vi "THD_MSA.vi"() -> ()   [LabVIEW 2012]
panel:
  out "Meas_Error":bool=TRUE
  in  "timeout(s)":dbl=10.0
  out "index":i32=48
  out "mean(THD)":dbl=0.5
  out "Sensitivity(mVeff/Pa)":dbl=336.0
  in  "Std_Deviation_Thresold":dbl=0.04
  in  "Excitation_amplitude(Vpeak)":dbl=0.35 min=0.0 format="%.3f"
  in  "Sound_Pressure(dB SPL)":dbl=94.0502
  in  "stop":bool=TRUE
  in  "Anzahl der Messungen":i32=200
  out "XY Graph":cluster{dbl[], dbl[]}[](graph)=[{[0.84, 0.944, 1.048, 1.1540000000000001, 1.2590000000000001, 1.3650000000000002, 1.4670000000000003, 1.5720000000000003, 1.6750000000000003, 1.7800000000000002, 1.8880000000000003, 1.9940000000000004, 2.0990000000000006, 2.206000000000001, 2.3080000000000007, 2.412000000000001, 2.520000000000001, 2.626000000000001, 2.733000000000001, 2.836000000000001, 2.942000000000001, 3.048000000000001, 3.154000000000001, 3.2600000000000007, 3.3640000000000008, 3.467000000000001, 3.573000000000001, 3.677000000000001, 3.783000000000001, 3.888000000000001, 3.9930000000000008, 4.099000000000001, 4.201000000000001, 4.307000000000001, 4.412000000000002, 4.517000000000002, 4.6220000000000026, 4.721000000000003, 4.827000000000003, 4.9330000000000025, 5.039000000000002, 5.1430000000000025, 5.248000000000003, 5.354000000000003, 5.461000000000003, 5.568000000000003, 5.674000000000003, 5.780000000000003, 5.885000000000003], [0.5, 0.5, 0.5, 0.5, 0.5, 0.5, 0.5, 0.5, 0.5, 0.5, 0.5, 0.5, 0.5, 0.5, 0.5, 0.5, 0.5, 0.5, 0.5, 0.5, 0.5, 0.5, 0.5, 0.5, 0.5, 0.5, 0.5, 0.5, 0.5, 0.5, 0.5, 0.5, 0.5, 0.5, 0.5, 0.5, 0.5, 0.5, 0.5, 0.5, 0.5, 0.5, 0.5, 0.5, 0.5, 0.5, 0.5, 0.5, 0.5]}, {[0.84, 0.944, 1.048, 1.1540000000000001, 1.2590000000000001, 1.3650000000000002, 1.4670000000000003, 1.5720000000000003, 1.6750000000000003, 1.7800000000000002, 1.8880000000000003, 1.9940000000000004, 2.0990000000000006, 2.206000000000001, 2.3080000000000007, 2.412000000000001, 2.520000000000001, 2.626000000000001, 2.733000000000001, 2.836000000000001, 2.942000000000001, 3.048000000000001, 3.154000000000001, 3.2600000000000007, 3.3640000000000008, 3.467000000000001, 3.573000000000001, 3.677000000000001, 3.783000000000001, 3.888000000000001, 3.9930000000000008, 4.099000000000001, 4.201000000000001, 4.307000000000001, 4.412000000000002, 4.517000000000002, 4.6220000000000026, 4.721000000000003, 4.827000000000003, 4.9330000000000025, 5.039000000000002, 5.1430000000000025, 5.248000000000003, 5.354000000000003, 5.461000000000003, 5.568000000000003, 5.674000000000003, 5.780000000000003, 5.885000000000003], [336.0, 336.0, 336.0, 336.0, 336.0, 336.0, 336.0, 336.0, 336.0, 336.0, 336.0, 336.0, 336.0, 336.0, 336.0, 336.0, 336.0, 336.0, 336.0, 336.0, 336.0, 336.0, 336.0, 336.0, 336.0, 336.0, 336.0, 336.0, 336.0, 336.0, 336.0, 336.0, 336.0, 336.0, 336.0, 336.0, 336.0, 336.0, 336.0, 336.0, 336.0, 336.0, 336.0, 336.0, 336.0, 336.0, 336.0, 336.0, 336.0]}, {[0.84, 0.944, 1.048, 1.1540000000000001, 1.2590000000000001, 1.3650000000000002, 1.4670000000000003, 1.5720000000000003, 1.6750000000000003, 1.7800000000000002, 1.8880000000000003, 1.9940000000000004, 2.0990000000000006, 2.206000000000001, 2.3080000000000007, 2.412000000000001, 2.520000000000001, 2.626000000000001, 2.733000000000001, 2.836000000000001, 2.942000000000001, 3.048000000000001, 3.154000000000001, 3.2600000000000007, 3.3640000000000008, 3.467000000000001, 3.573000000000001, 3.677000000000001, 3.783000000000001, 3.888000000000001, 3.9930000000000008, 4.099000000000001, 4.201000000000001, 4.307000000000001, 4.412000000000002, 4.517000000000002, 4.6220000000000026, 4.721000000000003, 4.827000000000003, 4.9330000000000025, 5.039000000000002, 5.1430000000000025, 5.248000000000003, 5.354000000000003, 5.461000000000003, 5.568000000000003, 5.674000000000003, 5.780000000000003, 5.885000000000003], [0.84, 0.104, 0.104, 0.106, 0.105, 0.106, 0.102, 0.105, 0.103, 0.105, 0.108, 0.106, 0.105, 0.107, 0.102, 0.104, 0.108, 0.106, 0.107, 0.103, 0.106, 0.106, 0.106, 0.106, 0.104, 0.103, 0.106, 0.104, 0.106, 0.105, 0.105, 0.106, 0.102, 0.106, 0.105, 0.105, 0.105, 0.099, 0.106, 0.106, 0.106, 0.104, 0.105, 0.106, 0.107, 0.107, 0.106, 0.106, 0.105]}]
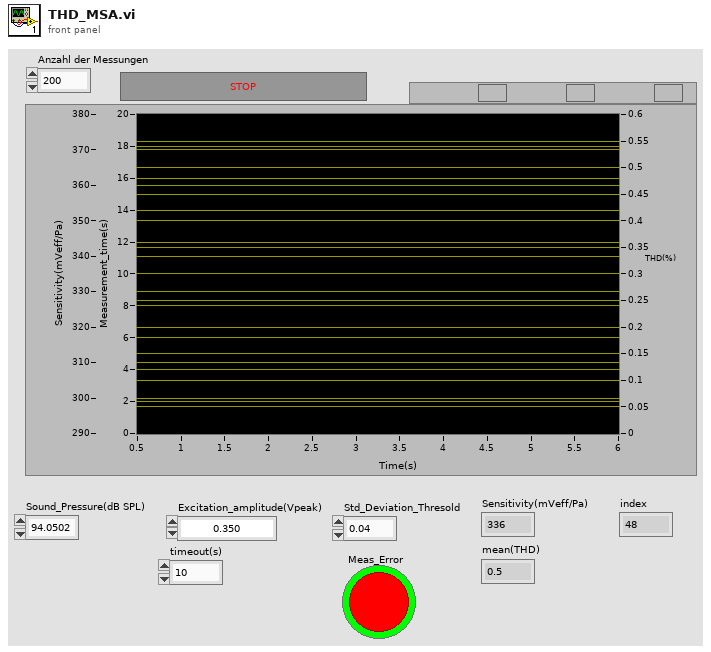
[diagram p1: front panel]
types:
  T1 = enum32{"Invalid", "Standard", "Closed", "Hidden", "Minimized", "Maximized"}
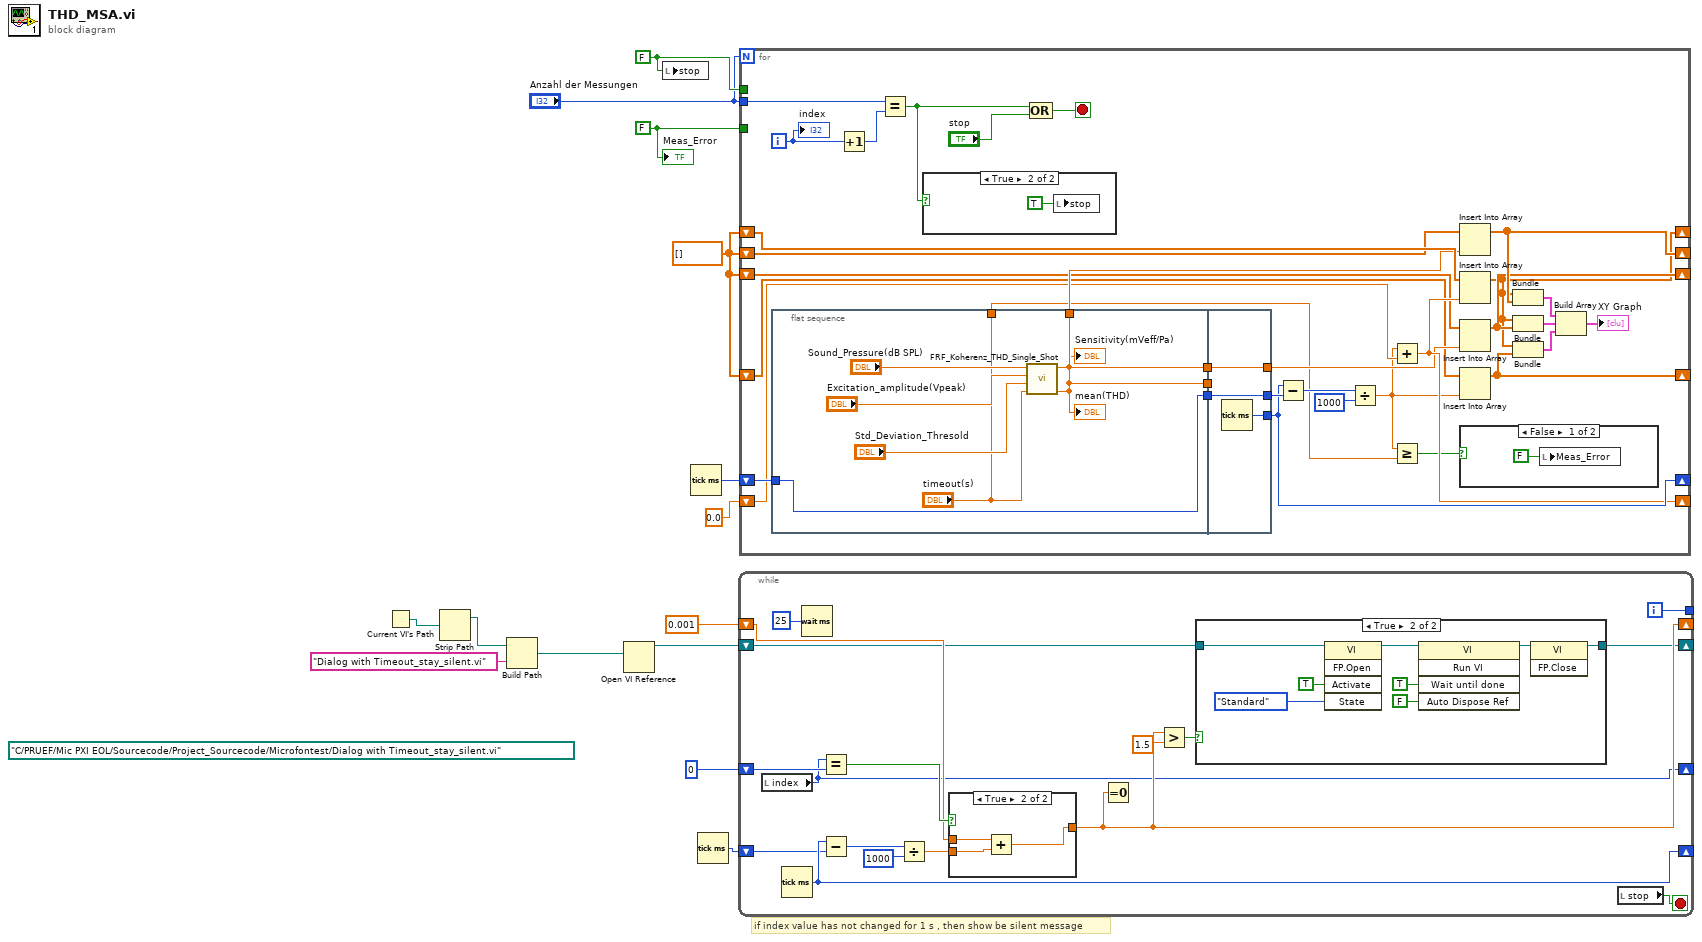
[diagram p0: block diagram]
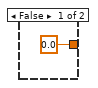
[diagram p3: hidden frame]
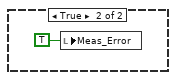
[diagram p4: hidden frame]
diagram:
  (unwired) path "C:/PRUEF/Mic PXI EOL/Sourcecode/Project_Sourcecode/Microfontest/Dialog with Timeout_stay_silent.vi" ("vi path")
  w5 = FALSE ("Meas_Error")
  w9 = FALSE ("stop")
  w6 = dbl[] []
  # "if index value has not changed for 1 s , then show be silent message"
  n1 = Current VI's Path() -> (path=w2:path)
  n2 = Strip Path(path=w2) -> (stripped path=w1:path)  [unwired: 1 out]
  n3 = Build Path(base path=w1, name or relative path="Dialog with Timeout_stay_silent.vi") -> (appended path=w3:path)
  n4 = Open VI Reference(vi path=w3) -> (vi reference=w7:refnum<vi>)  [unwired: 5 in, 1 out]
  n5 = local write "stop"(w9) -> ()
  n6 = Tick Count (ms)() -> (millisecond timer value=w14:u32)
  n7 = Tick Count (ms)() -> (millisecond timer value=w12:u32)
  n8 = while {
    shift-right: [w19] -> _
    shift-left: 0 ("index") -> [w31]
    shift-right: [w30] -> _
    shift-left: w12 -> [w29]
    shift-right: [w22] -> _
    shift-left: 0.001 -> [w25]
    tunnel: [w18] -> _
    shift-right: [w16] -> _
    shift-left: w7 -> [w17]
    i -> [w18]
    stop <- w21 stop-if-true
    n9 = local read "index"() -> (w19:i32)
    n10 = Tick Count (ms)() -> (millisecond timer value=w30:u32)
    n11 = Wait (ms)(milliseconds to wait=u32 25) -> ()  [unwired: 1 out]
    n12 = Equal?(x=w19, y=w31) -> (x = y?=w28:bool)
    n13 = Subtract(x=w30, y=w29) -> (x-y=w27:u32)
    n14 = Divide(x=w27, y=u32 1000) -> (x/y=w24:dbl)
    n15 = case shown="True" w28 {
      tunnel: w25 -> [_ w44]
      tunnel: w24 -> [_ w43]
      tunnel: [0.0 w42] -> w22
      frame False {
      }
      frame True {
        n16 = Add(x=w44, y=w43) -> (x+y=w42:dbl)
      }
    }
    n17 = Equal To 0?(x=w22) -> ()  [unwired: 1 out]
    n18 = Greater?(x=w22, y=1.5) -> (0:w15:bool)
    n19 = case shown="True" w15 {
      tunnel: w17 -> [w32 w36]
      tunnel: [w32 w33] -> w16
      frame False {
      }
      frame True {
        n20 = invoke class="VI" method="FP.Open"(reference=w36, "Activate"=TRUE ("Activate?"), "State"=T1."Standard") -> (reference out=w35:refnum<vi>)  [unwired: 2 in, 4 out]
        n21 = invoke class="VI" method="Run VI"(reference=w35, "Wait until done"=TRUE ("Wait Until Done"), "Auto Dispose Ref"=FALSE ("Auto Dispose Reference")) -> (reference out=w34:refnum<vi>)  [unwired: 2 in, 4 out]
        n22 = invoke class="VI" method="FP.Close"(reference=w34) -> (reference out=w33:refnum<vi>)  [unwired: 2 in, 2 out]
      }
    }
    n23 = local read "stop"() -> (w21:bool)
  }
  n24 = for {
    N: "Anzahl der Messungen" -> [_]
    shift-right: [w73] -> _
    shift-left: w14 -> [w76]
    shift-right: [w50] -> _
    shift-left: w6 -> [w70]
    shift-right: [w66] -> _
    shift-left: w6 -> [w67]
    shift-right: [w69] -> _
    shift-left: 0.0 -> [w51]
    shift-right: [w59] -> _
    shift-left: w6 -> [w63]
    tunnel: w9 -> [_]
    tunnel: "Anzahl der Messungen" -> [w56]
    shift-right: [w49] -> _
    shift-left: w6 -> [w52]
    tunnel: w5 -> [_]
    i -> [w58]
    stop <- w54 stop-if-true
    n25 = flat-sequence {
      tunnel: [w86] -> w77
      tunnel: w76 -> [w87]
      tunnel: [w87] -> w74
      tunnel: [w86] -> w68
      tunnel: [w84] -> w65
      tunnel: ["timeout(s)"] -> w45
      tunnel: w77 -> [_]
      tunnel: [w90] -> w73
      tunnel: [w89] -> w75
      tunnel: w74 -> [w89]
      tunnel: [w88] -> w64
      tunnel: w65 -> [w88]
      frame #0 {
        n26 = call "FRF_Koherenz_THD_Single_Shot.vi"("timeout(s)"="timeout(s)", "Std_Deviation_Thresold"="Std_Deviation_Thresold", "Excitation_amplitude(Vpeak)"="Excitation_amplitude(Vpeak)", "dB SPL"="Sound_Pressure(dB SPL)") -> ("mean"=w86:dbl, "Sensitivity(mVeff/Pa)"=w84:dbl)  [unwired: 5 in, 1 out]
        "Sensitivity(mVeff/Pa)" <- w84
        "mean(THD)" <- w86
      }
      frame #1 {
        n27 = Tick Count (ms)() -> (millisecond timer value=w90:u32)
      }
    }
    n28 = Increment(x=w58) -> (x+1=w57:i32)
    n29 = Equal?(x=w56, y=w57) -> (x = y?=w53:bool)
    n30 = case shown="True" w53 {
      frame False {
      }
      frame True {
        n31 = local write "stop"(TRUE ("stop")) -> ()
      }
    }
    n32 = Compound Arithmetic op=OR(w53, "stop") -> (w54:bool)
    n33 = Subtract(x=w73, y=w75) -> (x-y=w72:u32)
    n34 = Divide(x=w72, y=u32 1000) -> (x/y=w47:dbl)
    n35 = Add(x=w47, y=w51) -> (x+y=w69:dbl)
    n36 = Greater Or Equal?(x=w47, y=w45) -> (x >= y?=w46:bool)
    n37 = Insert Into Array(array=w67, new element=w68) -> (w66:dbl[])  [unwired: 1 in]
    n38 = Insert Into Array(array=w70, new element=w69) -> (w50:dbl[])  [unwired: 1 in]
    n39 = Insert Into Array(array=w63, new element=w64) -> (w59:dbl[])  [unwired: 1 in]
    n40 = Insert Into Array(array=w52, new element=w47) -> (w49:dbl[])  [unwired: 1 in]
    n41 = case shown="False" w46 {
      frame False {
        n42 = local write "Meas_Error"(FALSE ("Meas_Error")) -> ()
      }
      frame True {
        n43 = local write "Meas_Error"(TRUE ("Meas_Error")) -> ()
      }
    }
    n44 = Bundle(w50, w66) -> (w62:cluster{dbl[], dbl[]})  [unwired: 1 in]
    n45 = Bundle(w50, w59) -> (w61:cluster{dbl[], dbl[]})  [unwired: 1 in]
    n46 = Bundle(w50, w49) -> (w48:cluster{dbl[], dbl[]})  [unwired: 1 in]
    n47 = Build Array(w62, w61, w48) -> (→"XY Graph":cluster{dbl[], dbl[]}[])
    "index" <- w58
  }
  "Meas_Error" <- w5
